vi "ADIS16448_RoboRIO_Teensy_GetData.vi"(8 "error in":errorcluster, 11 "SerialPortRefIn":T2) -> (0 "error out":errorcluster, 1 "IMU AHRS Out":cluster{"Pitch":dbl, "Roll":dbl, "Yaw":dbl}, 2 "IMU Angles Out":T1, 3 "SerialPortRefOut":T2)   [LabVIEW 2016, in "ADIS16448-Teensy.lvlib"]
uses:
  ADIS16448-Teensy.lvlib
  <vilib>/Rock Robotics/WPI/SerialPort/WPI_SerialPortRef.ctl
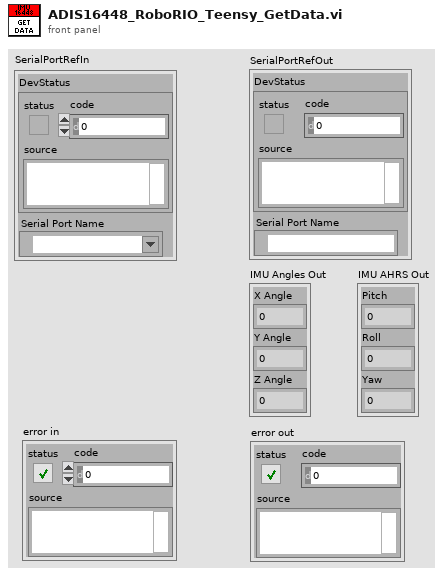
[diagram p1: front panel]
types:
  T1 = cluster{"X Angle":dbl, "Y Angle":dbl, "Z Angle":dbl}
  T2 = typedef "WPI_SerialPortRef.ctl" = cluster{"DevStatus":errorcluster, "Serial Port Name":refnum<visa-resource-name>}
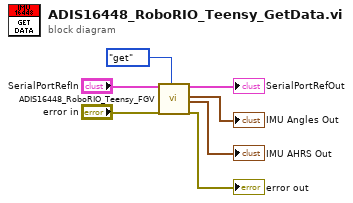
[diagram p0: block diagram]
diagram:
  n1 = call "ADIS16448_RoboRIO_Teensy_FGV.vi"("SerialPortRefIn"="SerialPortRefIn", "error in"="error in", "Operation"=enum16{"set", "get", "set reset"}."get") -> ("SerialPortRefOut"=→"SerialPortRefOut":T2, "IMU Angles Out"=→"IMU Angles Out":T1, "IMU AHRS Out"=→"IMU AHRS Out":cluster{"Pitch":dbl, "Roll":dbl, "Yaw":dbl}, "error out"=→"error out":errorcluster)  [unwired: 11 in, 2 out]
